vi "loop  filter.vi"(8 "g2":dbl, 9 "g1":dbl, 10 "in":dbl) -> (2 "out":dbl)   [LabVIEW 2017]
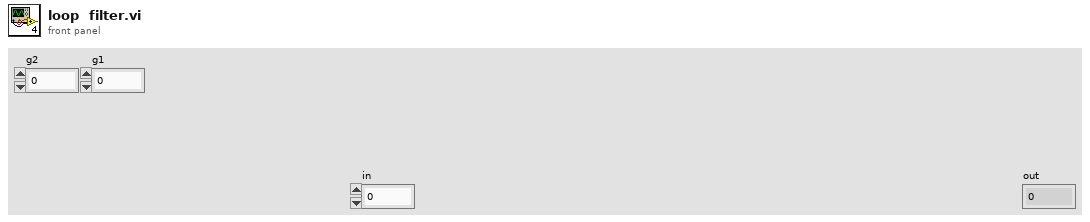
[diagram p1: front panel]
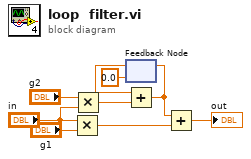
[diagram p0: block diagram]
diagram:
  n1 = Multiply(x="in", y="g1") -> (x*y=w8:dbl)
  n2 = Multiply(x="g2", y="in") -> (x*y=w9:dbl)
  n3 = feedback #1(0.0) -> (w6:dbl)
  n4 = Add(x=w6, y=w9) -> (x+y=w7:dbl)
  n5 = feedback-in #1(w7) -> ()
  n6 = Add(x=w7, y=w8) -> (x+y=→"out":dbl)
